vi "fromXML.vi"(8 "error in (no error)":errorcluster, 10 "xmlNode":refnum<class "xmlNode.lvclass">, 11 "HWConfiguration in":refnum<class "HWConfigurations.lvclass">) -> (0 "error out":errorcluster, 3 "HWConfiguration out":refnum<class "HWConfigurations.lvclass">)   [LabVIEW 2009, in "Tools.lvlib" / "DatabaseHelpers.lvlib" / "HWConfigurations.lvclass"]
uses:
  HWConfigurations.lvclass
  xmlNode/xmlNode.lvclass
  HWConfigurations.lvclass/HWConfigurations.ctl
  OutputConfiguration/OutputConfiguration.lvclass
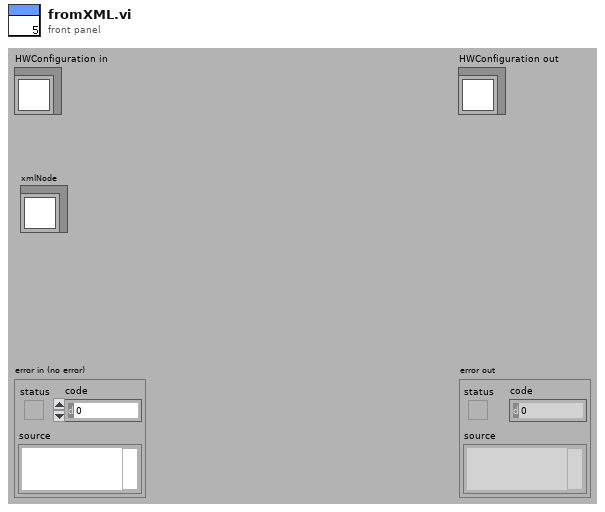
[diagram p1: front panel]
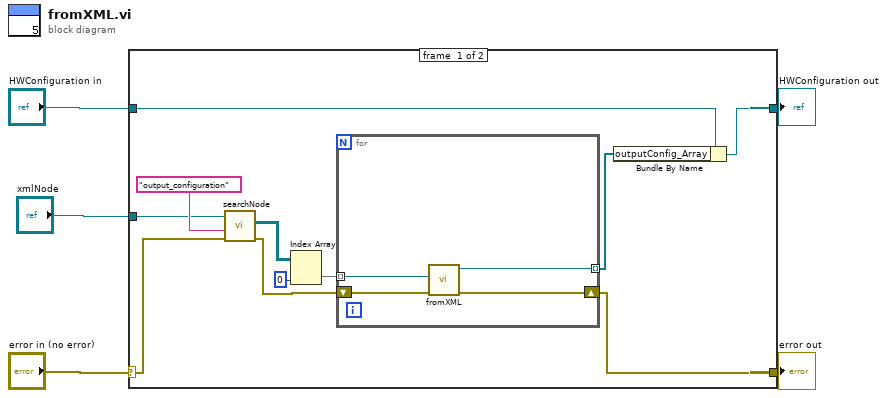
[diagram p0: block diagram]
diagram:
  n1 = case shown="No Error" "error in (no error)" {
    selector: "error in (no error)" -> [w11 w22]
    tunnel: [w9 w22] -> w4
    tunnel: [w6 w21] -> w2
    tunnel: "HWConfiguration in" -> [w7 w21]
    tunnel: "xmlNode" -> [w13 _]
    frame #0 {
      n2 = call-dynamic "searchNode.vi"("error in (no error)"=w11, "searchElementName"="output_configuration", "xmlNode in"=w13) -> ("error out"=w10:errorcluster, "arrayXmlNodes"=w15:refnum<class "xmlNode.lvclass">[][])  [unwired: 6 in, 1 out]
      n3 = Index Array(array=w15, index (col)=0) -> (element=w12:refnum<class "xmlNode.lvclass">[])  [unwired: 1 in]
      n4 = for {
        tunnel: w12 -> [w20] mode=indexing
        shift-right: [w18] -> w9
        shift-left: w10 -> [w19]
        tunnel: [w17] -> w8 mode=indexing
        n5 = call "fromXML.vi"("error in (no error)"=w19, "xmlNode"=w20) -> ("error out"=w18:errorcluster, "OutputConfiguration out"=w17:refnum<class "OutputConfiguration.lvclass">)  [unwired: 8 in]
      }
      n6 = Bundle By Name(cluster=w7, "outputConfig_Array"=w8) -> (w6:refnum<class "HWConfigurations.lvclass">)
    }
    frame #1 {
    }
  }
  "error out" <- w4
  "HWConfiguration out" <- w2
